vi "Change subscription count.vi"(8 "error in (no error)":errorcluster, 9 "Count change":i64, 10 "Topic":string, 11 "WAMP Client in":refnum<class "WAMP Client.lvclass">) -> (0 "error out":errorcluster, 3 "WAMP Client out":refnum<class "WAMP Client.lvclass">)   [LabVIEW 2020, in "wamplv.lvlib" / "WAMP Client.lvclass"]
uses:
  WAMP Client.lvclass
  WAMP Client.lvclass/WAMP Client.ctl
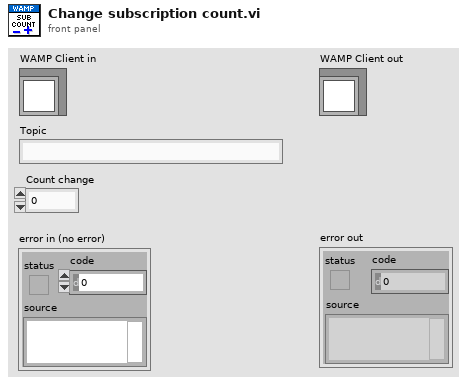
[diagram p1: front panel]
types:
  T1 = typedef "wamplv.lvlib/WAMP Client.lvclass/Message Loop Data.ctl" = cluster{"Last Request ID":u64, "Register Requests":map{u64, T2}, "Publish Requests":T3, "Endpoints Map":map{u64, T5}, "Call Requests":T6, "Subscription Requests":T8, "Subscriptions":T10, "Unsubscribe Requests":T12, "Random Request IDs":u64[], "Unregister requests map":T14}
  T2 = typedef "wamplv.lvlib/WAMP Client.lvclass/REGISTER Request Data.ctl" = cluster{"Procedure URI":string, "Options":string, "REGISTER result notifier":refnum<notifier>}
  T3 = typedef "wamplv.lvlib/WAMP Client.lvclass/Publish Requests Map.ctl" = map{u64, T4}
  T4 = typedef "wamplv.lvlib/WAMP Client.lvclass/PUBLISH Request Data.ctl" = cluster{"Topic URI":string, "Arguments":string, "ArgumentsKw":string, "Request Acknowledgement":bool, "Options":string, "Publish result notifier":refnum<notifier>}
  T5 = typedef "wamplv.lvlib/WAMP Client.lvclass/Endpoint Data.ctl" = cluster{"Procedure URI":string}
  T6 = typedef "wamplv.lvlib/WAMP Client.lvclass/CALL Request Map.ctl" = map{u64, T7}
  T7 = typedef "wamplv.lvlib/WAMP Client.lvclass/CALL Request Data.ctl" = cluster{"Topic URI":string, "Arguments":string, "ArgumentsKw":string, "Options":string, "Call result":refnum<notifier>}
  T8 = typedef "wamplv.lvlib/WAMP Client.lvclass/SUBSCRIBE Requests Map.ctl" = map{u64, T9}
  T9 = typedef "wamplv.lvlib/WAMP Client.lvclass/SUBSCRIBE Request Data.ctl" = cluster{"Topic":string, "Subscribe result notifer":refnum<notifier>, "Options":string}
  T10 = typedef "wamplv.lvlib/WAMP Client.lvclass/Subscriptions Map.ctl" = map{u64, T11}
  T11 = typedef "wamplv.lvlib/WAMP Client.lvclass/Subscription Details.ctl" = cluster{"Subscription ID":u64, "Topic":string, "Publication Received Event":refnum<user-event>, "Publication Received Notifier":refnum<notifier>, "Number of subscriptions":u64}
  T12 = typedef "wamplv.lvlib/WAMP Client.lvclass/Unsubscribe Requests Map.ctl" = map{u64, T13}
  T13 = typedef "wamplv.lvlib/WAMP Client.lvclass/UNSUBSCRIBE Request Data.ctl" = cluster{"Topic":string, "Unsubscrube result notifier":refnum<notifier>, "Options":string}
  T14 = typedef "wamplv.lvlib/WAMP Client.lvclass/Unregister requests map.ctl" = map{u64, T15}
  T15 = typedef "wamplv.lvlib/WAMP Client.lvclass/Unregister request.ctl" = cluster{"URI":string, "Unregister result notifier":refnum<notifier>, "Options":string}
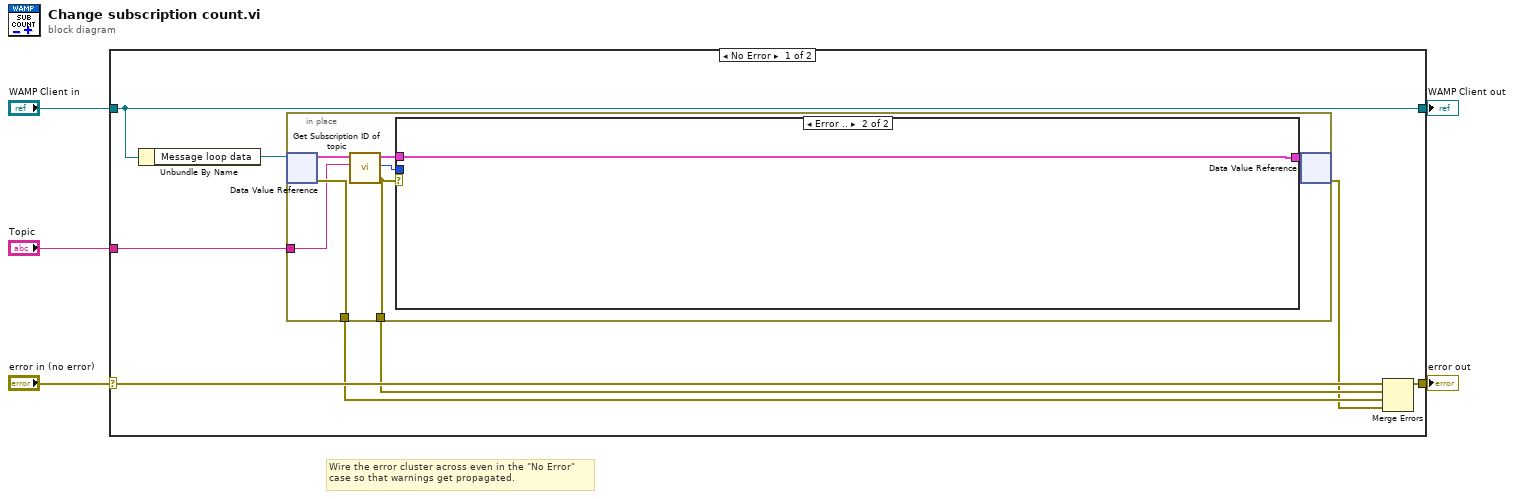
[diagram p0: block diagram]
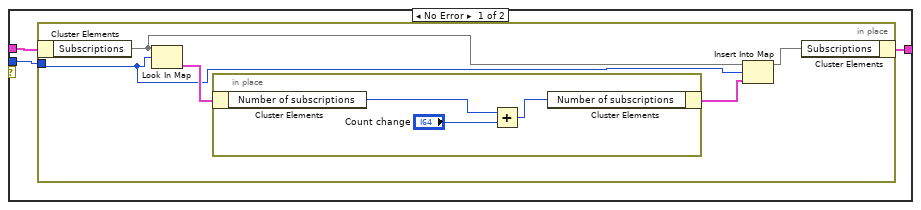
[diagram p2: hidden frame]
diagram:
  # "Wire the error cluster across even in the \"No Error\"\ncase so that warnings get propagated."
  n1 = case shown="No Error" "error in (no error)" {
    selector: "error in (no error)" -> [w10 w34]
    tunnel: [w9 w34] -> w4
    tunnel: [w13 w33] -> w2
    tunnel: "WAMP Client in" -> [w13 w33]
    tunnel: "Topic" -> [w11 _]
    frame No Error {
      n2 = Unbundle By Name(w13) -> ("Message loop data"=w12:refnum<data-value>)
      n3 = in-place {
        in-place-border: w11 -> [w18]
        in-place-border: [w19] -> w8
        in-place-border: [w14] -> w7
        n4 = in-place-dvr #1(w12) -> (w20:T1, w19:errorcluster)
        n5 = call "Get Subscription ID of topic.vi"("Topic"=w18, "Message loop data (in)"=w20) -> ("error out"=w14:errorcluster, "Subscription ID"=w16:u64, "Message loop data (out)"=w17:T1)  [unwired: 7 in]
        n6 = case shown="Error .." w14 {
          tunnel: w17 -> [w23 w32]
          tunnel: w16 -> [w22 _]
          tunnel: [w21 w32] -> w15
          frame No Error {
            n7 = in-place {
              in-place-border: w22 -> [w25]
              n8 = in-place-cluster #2(w23) -> ("Subscriptions"=w27:T10)
              n9 = Look In Map(map=w27, key=w25) -> (value=w28:T11)  [unwired: 1 in, 1 out]
              n10 = in-place {
                n11 = in-place-cluster #3(w28) -> ("Number of subscriptions"=w31:u64)
                n12 = Add(x=w31, y="Count change") -> (x+y=w29:u64)
                n13 = in-place-cluster #3("Number of subscriptions"=w29) -> (w26:T11)
              }
              n14 = Insert Into Map(map in=w27, key=w25, value=w26) -> (map out=w24:T10)  [unwired: 2 out]
              n15 = in-place-cluster #2("Subscriptions"=w24) -> (w21:T1)
            }
          }
          frame Error {
          }
        }
        n16 = in-place-dvr #1(w15) -> (w6:errorcluster)  [unwired: 1 out]
      }
      n17 = Merge Errors(w10, w7, w8, w6) -> (w9:errorcluster)
    }
    frame Error {
    }
  }
  "error out" <- w4
  "WAMP Client out" <- w2
